vi "בדיקת זמן מיתוג הממסר 4.vi"(7 "resultUserPrompt":bool, 8 "error":errorcluster, 11 "Path for Log":path) -> (0 "error out":errorcluster, 1 "בטוח כן/לא":bool, 2 "בדיקת זמן מיתוג הממסר":dbl)   [LabVIEW 2014]
uses:
  <instrlib>/niDMM/nidmm.llb/niDMM Function.ctl
  <instrlib>/niDMM/nidmm.llb/niDMM Resolution in Digits.ctl
  <vilib>/DAQmx/create/channels.llb/DAQmx Create Channel (DO-Digital Output).vi
  <instrlib>/niDMM/nidmm.llb/niDMM Configure Measurement Digits.vi
  <vilib>/DAQmx/write.llb/DAQmx Write (Digital Bool 1Line 1Point).vi
panel:
  in  "התחל":bool
  # "Right-Click to\nexplain error"
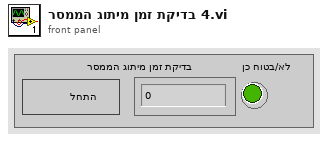
[diagram p1: front panel]
types:
  T1 = enum32{"Invalid", "Standard", "Closed", "Hidden", "Minimized", "Maximized"}
  T2 = typedef "niDMM Function.ctl" = enum16{"DC Volts", "AC Volts", "DC Current", "AC Current", "2-wire Resistance", "4-wire Resistance", "Diode", "Frequency", "Period", "AC Volts DC Coupled", "Capacitance", "Inductance", "Temperature"}
  T3 = typedef "niDMM Resolution in Digits.ctl" = dbl
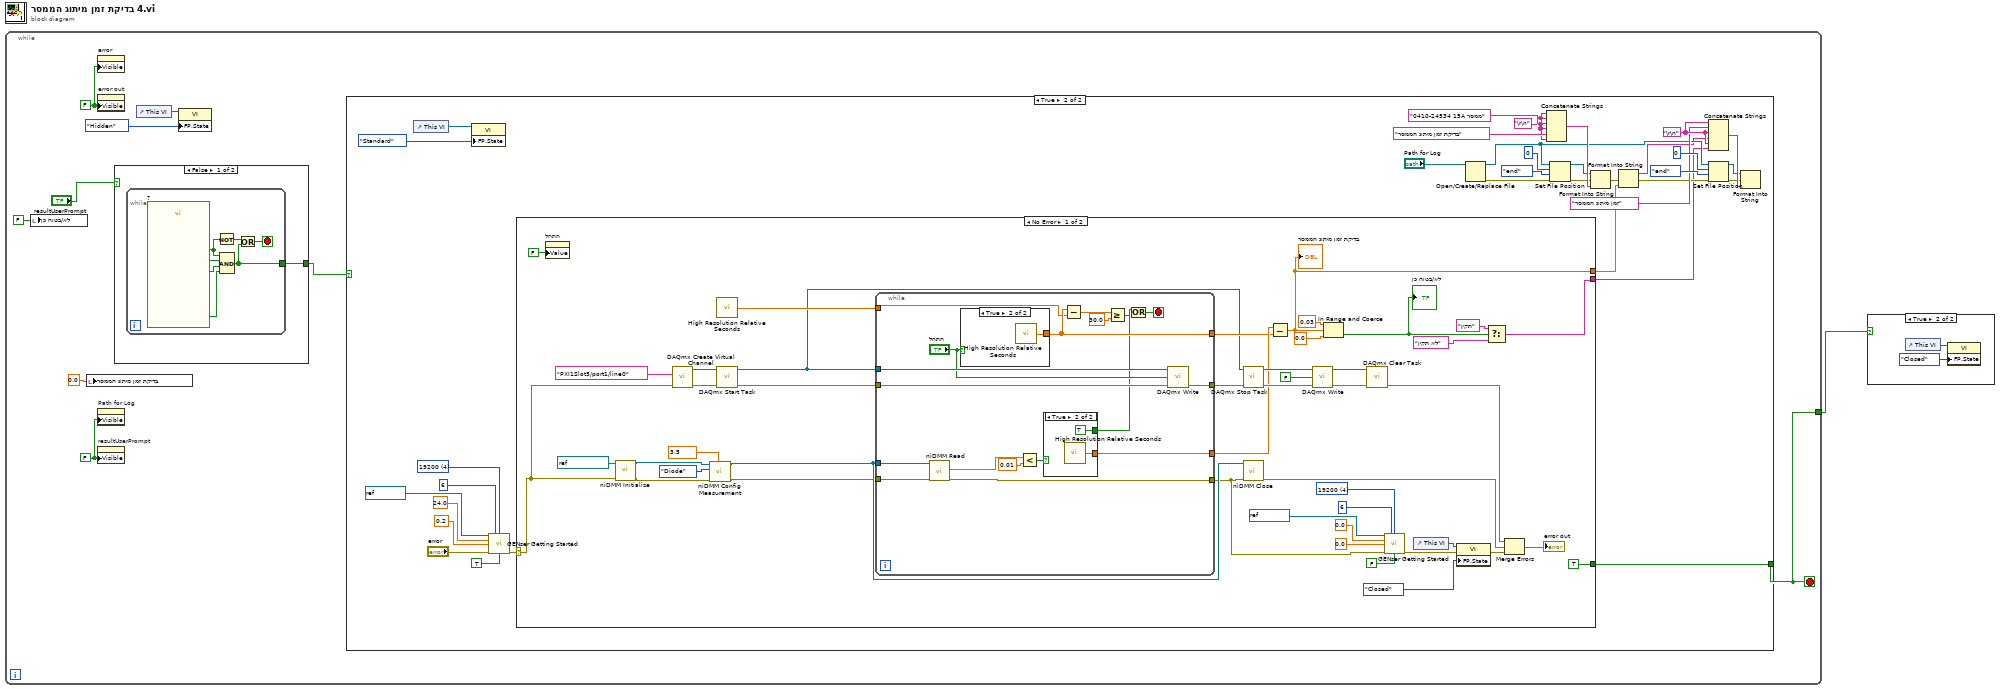
[diagram p0: block diagram]
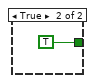
[diagram p3: hidden frame]
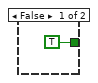
[diagram p4: hidden frame]
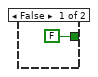
[diagram p5: hidden frame]
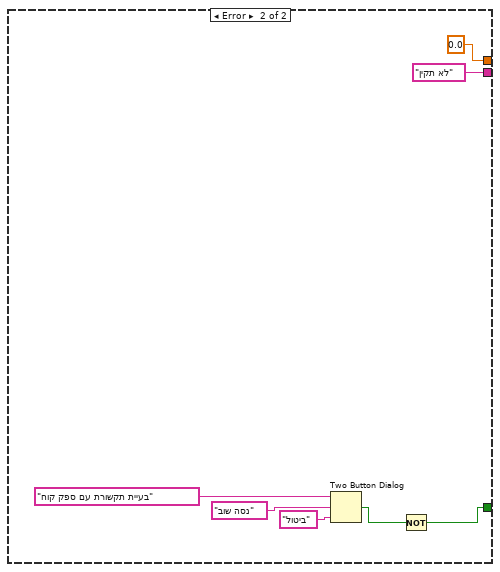
[diagram p7: hidden frame]
diagram:
  n1 = while {
    tunnel: [w2] -> w1
    stop <- w2 stop-if-true
    w3 = FALSE ("Visible")
    w10 = FALSE ("Visible")
    n2 = local write "בטוח כן/לא"(FALSE ("בטוח כן/לא")) -> ()
    n3 = local write "בדיקת זמן מיתוג הממסר"(0.0 ("בדיקת זמן מיתוג הממסר")) -> ()
    n4 = property on="error" class="Clust (strict)"("Visible"=w10) -> ()  [unwired: 2 in, 2 out]
    n5 = property on="error out" class="Clust (strict)"("Visible"=w10) -> ()  [unwired: 2 in, 2 out]
    n6 = property on="Path for Log" class="Path"("Visible"=w3) -> ()  [unwired: 2 in, 2 out]
    n7 = property on="resultUserPrompt" class="Bool (strict)"("Visible"=w3) -> ()  [unwired: 2 in, 2 out]
    n8 = case shown="False" "resultUserPrompt" {
      tunnel: [w11 TRUE] -> w7
      frame False {
        n9 = while {
          tunnel: [w12] -> w11
          stop <- w15 stop-if-true
          n10 = call "?"() -> ("הדקי הרב מודד"=w16:bool, "(מגע שלילי (מעטפת"=w17:bool, "A מגע חיובי"=w18:bool, "OK"=w13:bool)  [unwired: 15 in, 1 out]
          n11 = Not(x=w13) -> (.not. x?=w14:bool)
          n12 = Compound Arithmetic op=AND(w13, w18, w17, w16) -> (w12:bool)
          n13 = Or(x=w14, y=w12) -> (x .or. y?=w15:bool)
        }
      }
      frame True {
      }
    }
    n14 = control-ref of="This VI"() -> (w9:refnum<vi>)
    n15 = property class="VI"(reference=w9, "FP.State"=T1."Hidden" ("Front Panel Window:State")) -> ()  [unwired: 1 in, 2 out]
    n16 = case shown="True" w7 {
      tunnel: [TRUE ("T button?") w47] -> w2
      frame False {
      }
      frame True {
        w30 = "\r\n"
        w37 = "\r\n"
        w50 = u16 4 items=["1200", "2400", "4800", "9600", "19200"] ("BAUD")
        n17 = control-ref of="This VI"() -> (w46:refnum<vi>)
        n18 = property class="VI"(reference=w46, "FP.State"=T1."Standard" ("Front Panel Window:State")) -> ()  [unwired: 1 in, 2 out]
        n19 = call "GENser Getting Started.vi"("VISA"=refnum<visa-resource-name> "COM6", "GEN Addr"=i16 6, "BAUD"=w50, "Voltage Limit"=24.0, "Current Limit"=0.2, "error"="error", "Output On (T)"=TRUE) -> ("error out"=w52:errorcluster)  [unwired: 5 in, 3 out]
        n20 = case shown="No Error" w52 {
          selector: w52 -> [w61 _]
          tunnel: [TRUE ("T button?") w122] -> w47
          tunnel: [w75 0.0] -> w22
          tunnel: [w71 "לא תקין"] -> w21
          frame No Error {
            w64 = T3 3.5 items=["3 1/2"=3.5, "4 1/2"=4.5, "5 1/2"=5.5, "6 1/2"=6.5, "7 1/2"=7.5] ("Resolution in Digits")
            w93 = u16 4 items=["1200", "2400", "4800", "9600", "19200"] ("BAUD")
            n21 = property on="התחל" class="Bool (strict)"("Value"=FALSE ("data")) -> ()  [unwired: 2 in, 2 out]
            n22 = call <instrlib>:"niDMM Initialize.vi"("error in (no error)"=w61, "Instrument Descriptor"=refnum<k15> "PXI1Slot9") -> ("error out"=w62:errorcluster, "instrument handle out"=w63:refnum<k15>)  [unwired: 8 in]
            n23 = call-poly <vilib>:"DAQmx Create Virtual Channel.vi"("lines"=tag "PXI1Slot5/port1/line0", "error in"=w61) -> ("task out"=w68:refnum<k21>, "error out"=w69:errorcluster)  [unwired: 12 in]
            n24 = call-poly <instrlib>:"niDMM Config Measurement.vi"("Resolution in Digits"=w64, "error in (no error)"=w62, "Function"=niDMM_Function."Diode", "instrument handle"=w63) -> ("error out"=w58:errorcluster, "instrument handle out"=w60:refnum<k15>)  [unwired: 6 in]
            n25 = call <vilib>:"High Resolution Relative Seconds.vi"() -> ("relative seconds"=w66:dbl)
            n26 = call <vilib>:"DAQmx Start Task.vi"("task/channels in"=w68, "error in"=w69) -> ("task out"=w59:refnum<k21>, "error out"=w57:errorcluster)  [unwired: 12 in]
            n27 = while {
              tunnel: [w111] -> w82
              tunnel: [w117] -> w83
              tunnel: w59 -> [w116]
              tunnel: w57 -> [w115]
              tunnel: w66 -> [w110]
              tunnel: w60 -> [w103]
              tunnel: w58 -> [w102]
              tunnel: [w101] -> w56
              tunnel: [w100] -> w55
              stop <- w107 stop-if-true
              n28 = call <instrlib>:"niDMM Read.vi"("error in (no error)"=w102, "instrument handle"=w103) -> ("error out"=w100:errorcluster, "Measurement"=w114:dbl)  [unwired: 7 in, 1 out]
              n29 = case shown="True" "התחל" {
                tunnel: [_ w121] -> w111
                frame False {
                }
                frame True {
                  n30 = call <vilib>:"High Resolution Relative Seconds.vi"() -> ("relative seconds"=w121:dbl)
                }
              }
              n31 = Less?(x=w114, y=0.01) -> (x < y?=w104:bool)
              n32 = case shown="True" w104 {
                tunnel: [_ w120] -> w117
                tunnel: [FALSE TRUE] -> w106
                frame False {
                }
                frame True {
                  n33 = call <vilib>:"High Resolution Relative Seconds.vi"() -> ("relative seconds"=w120:dbl)
                }
              }
              n34 = Subtract(x=w111, y=w110) -> (x-y=w109:dbl)
              n35 = Greater Or Equal?(x=w109, y=30.0) -> (x >= y?=w105:bool)
              n36 = Or(x=w106, y=w105) -> (x .or. y?=w107:bool)
              n37 = call-poly <vilib>:"DAQmx Write.vi"("task/channels in"=w116, "data"="התחל", "error in"=w115) -> ("error out"=w101:errorcluster)  [unwired: 10 in, 2 out]
            }
            n38 = call <vilib>:"DAQmx Stop Task.vi"("task/channels in"=w59, "error in"=w56) -> ("task out"=w88:refnum<k21>, "error out"=w87:errorcluster)  [unwired: 12 in]
            n39 = call <instrlib>:"niDMM Close.vi"("error in (no error)"=w55, "instrument handle"=w60) -> ("error out"=w79:errorcluster)  [unwired: 9 in]
            n40 = Subtract(x=w83, y=w82) -> (x-y=w75:dbl)
            "בדיקת זמן מיתוג הממסר" <- w75
            n41 = call-poly <vilib>:"DAQmx Write.vi"("task/channels in"=w88, "data"=FALSE, "error in"=w87) -> ("task out"=w85:refnum<k21>, "error out"=w86:errorcluster)  [unwired: 10 in, 1 out]
            n42 = In Range and Coerce(upper limit=0.03, x=w75, lower limit=0.0) -> (In Range?=w72:bool)  [unwired: 1 out]
            "בטוח כן/לא" <- w72
            n43 = call <vilib>:"DAQmx Clear Task.vi"("task in"=w85, "error in"=w86) -> ("error out"=w80:errorcluster)  [unwired: 13 in]
            n44 = call "GENser Getting Started.vi"("VISA"=refnum<visa-resource-name> "COM6", "GEN Addr"=i16 6, "BAUD"=w93, "Voltage Limit"=0.0, "Current Limit"=0.0, "error"=w55, "Output On (T)"=FALSE) -> ("error out"=w92:errorcluster)  [unwired: 5 in, 3 out]
            n45 = control-ref of="This VI"() -> (w91:refnum<vi>)
            n46 = property class="VI"(reference=w91, error in=w92, "FP.State"=T1."Closed" ("Front Panel Window:State")) -> (error out=w78:errorcluster)  [unwired: 1 out]
            n47 = Select(t="תקין", s=w72, f="לא תקין") -> (s? t:f=w71:string)
            n48 = Merge Errors(w80, w79, w78) -> (→"error out":errorcluster)
          }
          frame Error {
            n49 = Two Button Dialog(message="בעיית תקשורת עם ספק קוח", 1:"ביטול" ("F button name (\"Cancel\")"), 2:"נסה שוב" ("T button name (\"OK\")")) -> (T button?=w123:bool)
            n50 = Not(x=w123) -> (.not. x?=w122:bool)
          }
        }
        n51 = Open/Create/Replace File(file path (use dialog)="Path for Log") -> (refnum out=w26:refnum<file>, error out=w27:errorcluster)  [unwired: 5 in, 1 out]
        n52 = Concatenate Strings(w37, w37, "0410-24534 15A ממסר", w37, "בדיקת זמן מיתוג הממסר", w37) -> (w41:string)
        n53 = Set File Position(offset (in bytes) (0)=i64 0, refnum=w26, from (0:start)=enum16{"start", "end", "current"}."end", error in=w27) -> (refnum out=w38:refnum<file>, error out=w36:errorcluster)
        n54 = Format Into String(initial string=w38, error in=w36, w41) -> (error out=w25:errorcluster)  [unwired: 1 in, 1 out]
        n55 = Format Into String(error in=w25, w22) -> (resulting string=w23:string, error out=w24:errorcluster)  [unwired: 2 in]
        n56 = Concatenate Strings(w30, "זמן מיתוג הממסר", w30, w23, w30, w21) -> (w35:string)
        n57 = Set File Position(offset (in bytes) (0)=i64 0, refnum=w26, from (0:start)=enum16{"start", "end", "current"}."end", error in=w24) -> (refnum out=w33:refnum<file>, error out=w34:errorcluster)
        n58 = Format Into String(initial string=w33, error in=w34, w35) -> ()  [unwired: 1 in, 2 out]
      }
    }
  }
  n59 = case shown="True" w1 {
    frame False {
    }
    frame True {
      n60 = control-ref of="This VI"() -> (w129:refnum<vi>)
      n61 = property class="VI"(reference=w129, "FP.State"=T1."Closed" ("Front Panel Window:State")) -> ()  [unwired: 1 in, 2 out]
    }
  }
